vi "Set Extension.vi"(8 "error in (no error)":errorcluster, 11 "TXT_Report":refnum<class "TXT Report.lvclass">) -> (0 "error out":errorcluster, 3 "TXT_Report out":refnum<class "TXT Report.lvclass">)   [LabVIEW 2009, in "TXT Report.lvclass"]
doc: "This is a dynamic dispatch VI that defines the extension of .TXT for the object data that will be written to the file.\n\nAAL 9/09"
uses:
  TXT Report.lvclass
  Report Class/Report.lvclass
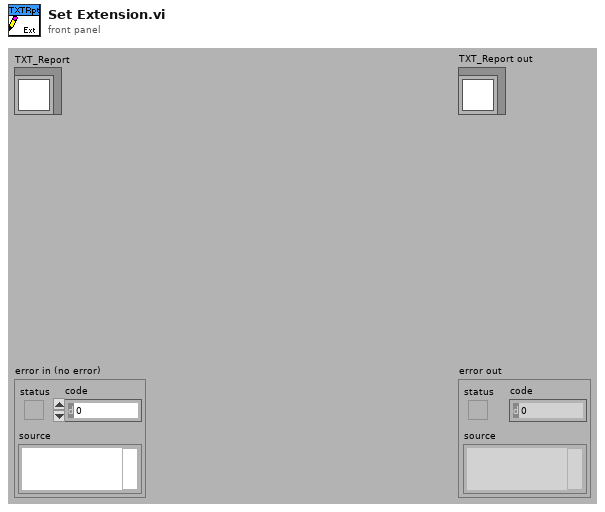
[diagram p1: front panel]
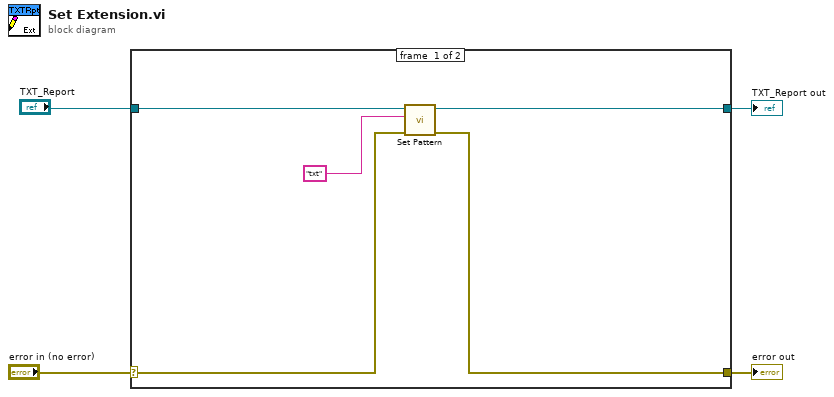
[diagram p0: block diagram]
diagram:
  n1 = case shown="Error" "error in (no error)" {
    selector: "error in (no error)" -> [w7 w11]
    tunnel: [w6 w11] -> w3
    tunnel: [w9 w10] -> w2
    tunnel: "TXT_Report" -> [w5 w10]
    frame #0 {
      n2 = call "Set Pattern.vi"("error in (no error)"=w7, "Pattern"="txt", "Report"=w5) -> ("error out"=w6:errorcluster, "Report out"=w9:refnum<class "TXT Report.lvclass">)  [unwired: 7 out]
    }
    frame #1 {
    }
  }
  "error out" <- w3
  "TXT_Report out" <- w2
